vi "Command.vi"(8 "error in (no error)":errorcluster, 11 "Node Ptr":T1 format="%.0x") -> (0 "error out":errorcluster)   [LabVIEW 2018, in "Instrument Addon System Explorer.lvlib"]
uses:
  Instrument Addon System Explorer.lvlib
  <vilib>/NI Veristand/Custom Device API/Custom Device Item Ref.ctl
  APIs/Scripting API/TypeDefs/Command Settings.ctl
  APIs/Scripting API/TypeDefs/Padding.ctl
  APIs/Scripting API/TypeDefs/Linked Channel.ctl
  Addon Shared/Types/Linked Channel Cluster.ctl
  Addon Shared/SubVIs/Constants.vi
  <vilib>/Utility/file.llb/Write Delimited Spreadsheet (string).vi
  <vilib>/NI VeriStand/Custom Device API/Custom Device API.lvlib
  Addon Shared/Instrument Addon Shared.lvlib
  APIs/Scripting API/Instrument Addon Scripting API.lvlib
panel:
  in  "Pad Value":u8=32 format="%.0x"
  in  "Length":u32=25 caption="Length (Bytes)"
  in  "Pad":bool caption="Pad?"
  in  "Linkages":i32(listbox)
  in  "MetaData":string(combo) caption="Available MetaData Channels"
  in  "Command":string caption="Command ( Use [] to define a variable )"
  in  "Header 2":cluster{"Section Name":string}={"Section Name"="Command Message Settings"}
  in  "SHDocVw.IWebBrowser":refnum<k7>(container)
  in  "Header":cluster{"Section Name":string}={"Section Name"="Command Settings"}
  in  "Description":string
  out "Name":string
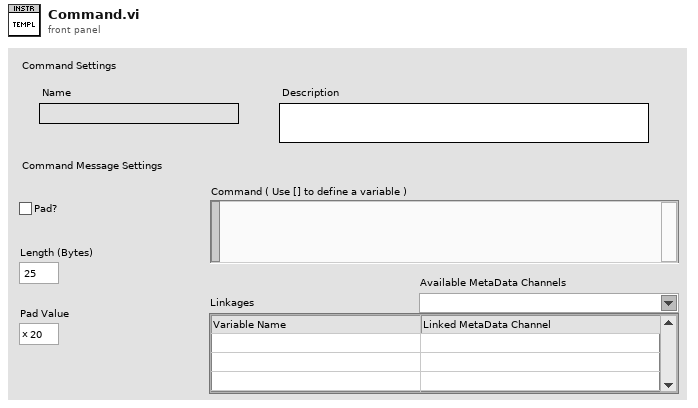
[diagram p1: front panel]
types:
  T1 = typedef "Custom Device API.lvlib/Custom Device Item Ref.ctl" = u64
  T2 = typedef "Instrument Addon Scripting API.lvlib/Command Settings.ctl" = cluster{"Command Format":string, "Use Padding?":bool, "Padding":T3, "Linkages":T4}
  T3 = typedef "Instrument Addon Scripting API.lvlib/Padding.ctl" = cluster{"Length":u32, "Pad Value":u8}
  T4 = typedef "Instrument Addon Scripting API.lvlib/Linked Channel.ctl" = cluster{"Channel Ref":T1, "Variable Name":string}[]
  T5 = typedef "Instrument Addon Shared.lvlib/Linked Channel Cluster.ctl" = cluster{"Variable Name":string, "GUID":string}
  T6 = cluster{"Channel Ref":T1, "Variable Name":string}
  T7 = typedef "Custom Device API.lvlib/Custom Device Item Info.ctl" = cluster{"Name":string, "Is Channel":bool, "GUID":string, "Is Waveform":bool}
  T8 = typedef "Custom Device API.lvlib/Custom Device Commands.ctl" = enum16{"Default", "Item renamed", "Shutdown", "Dynamic button pressed"}
  T9 = typedef "LVComboBoxStrsAndValuesArrayTypeDef.ctl" = cluster{"String":string, "Value":string}[]
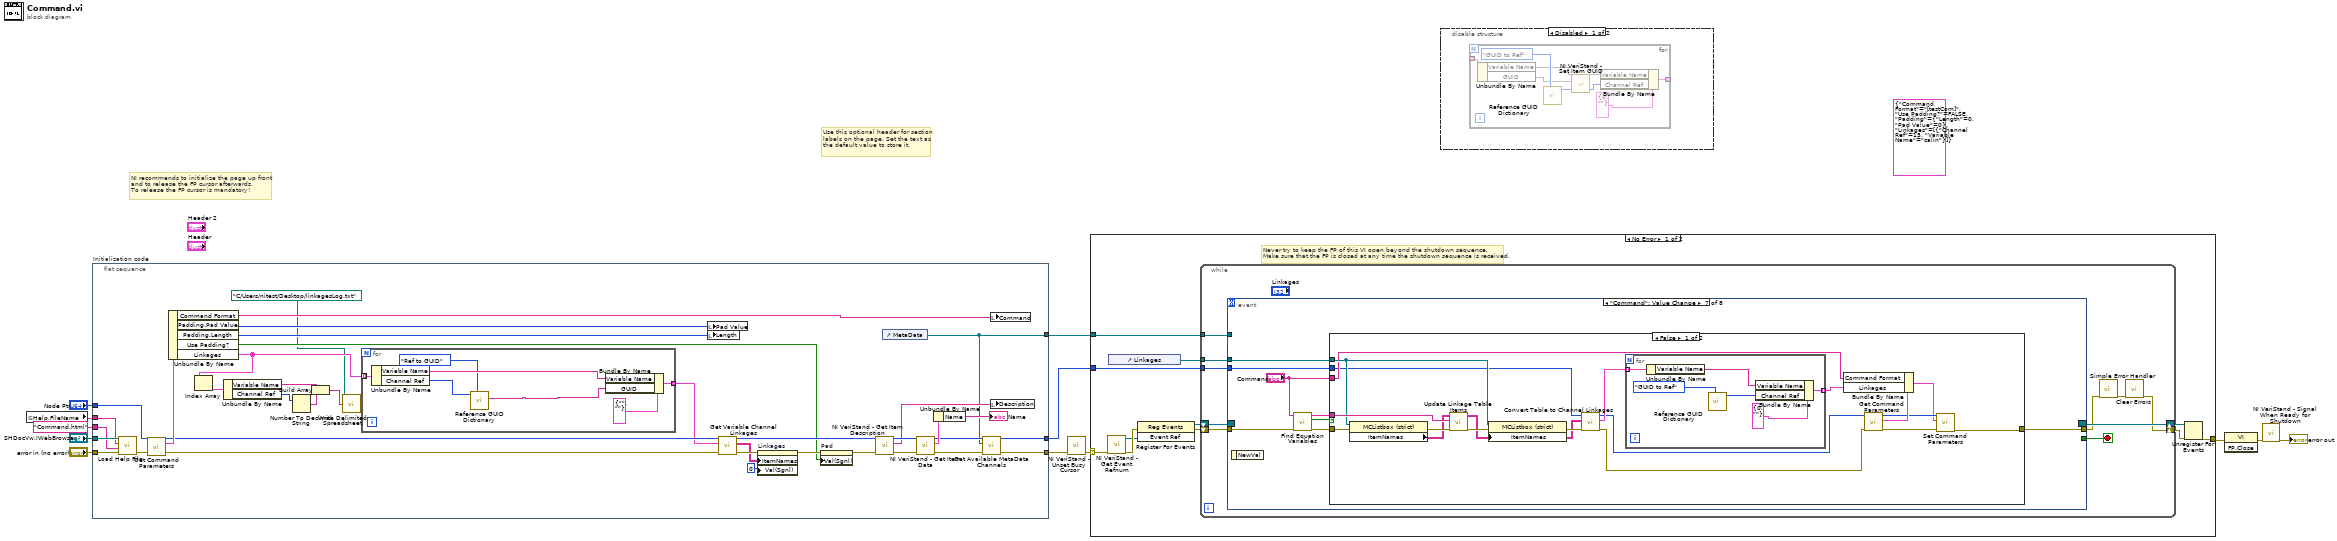
[diagram p0: block diagram]
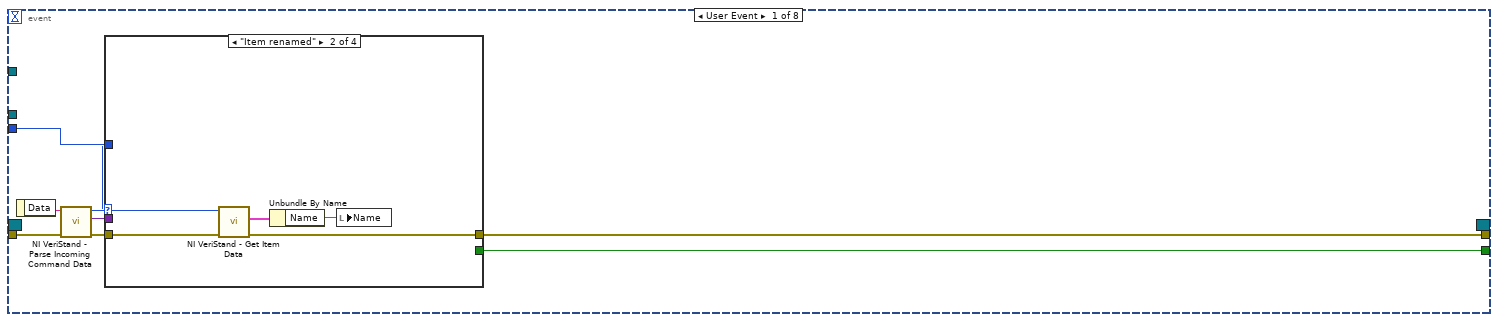
[diagram p3: hidden frame]
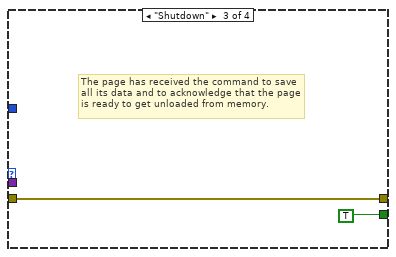
[diagram p5: hidden frame]
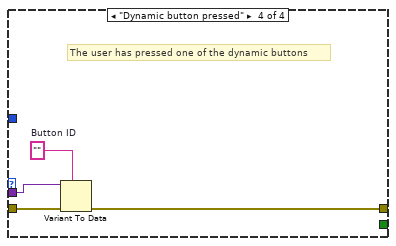
[diagram p6: hidden frame]
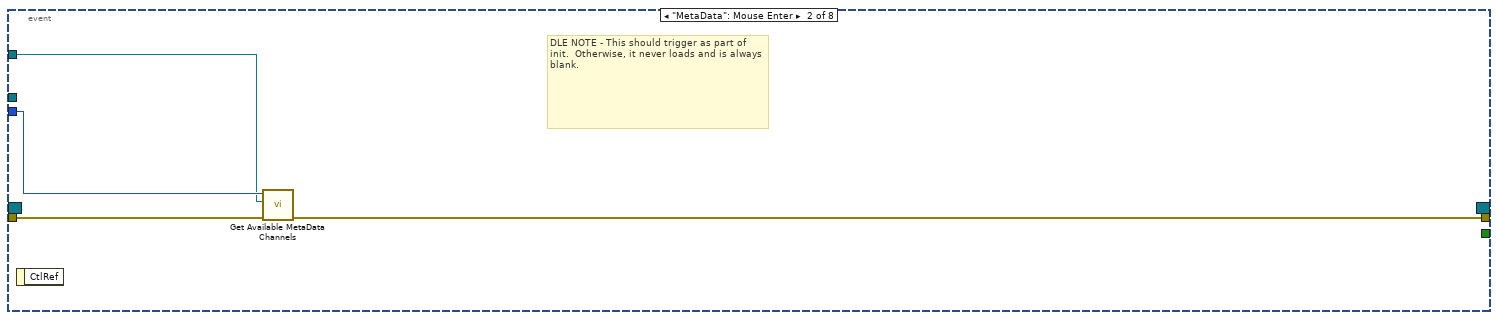
[diagram p7: hidden frame]
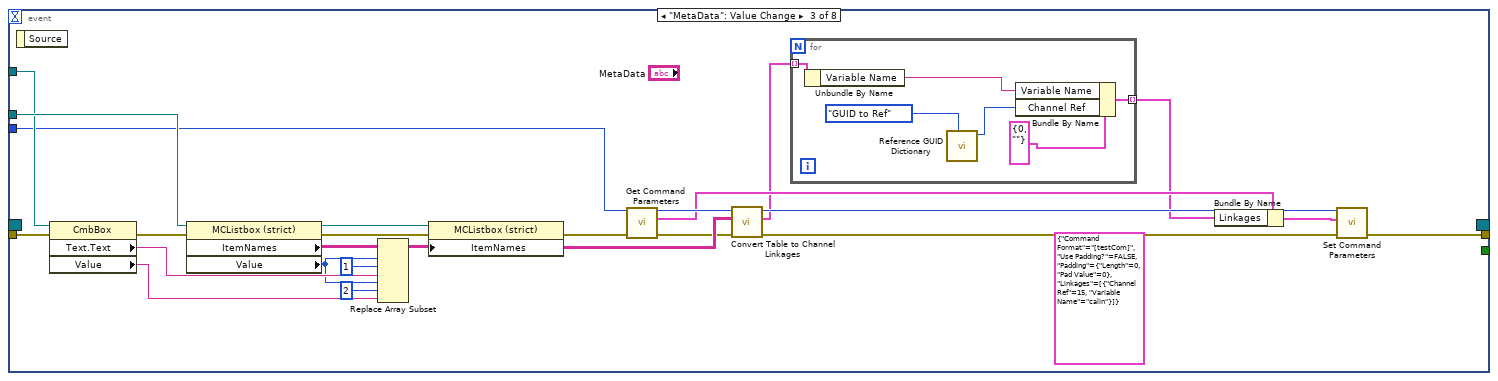
[diagram p8: hidden frame]
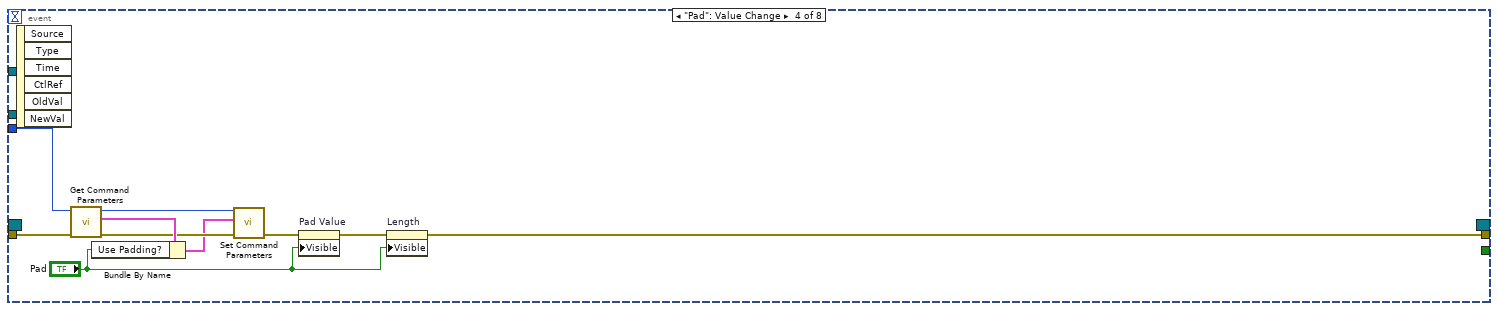
[diagram p9: hidden frame]
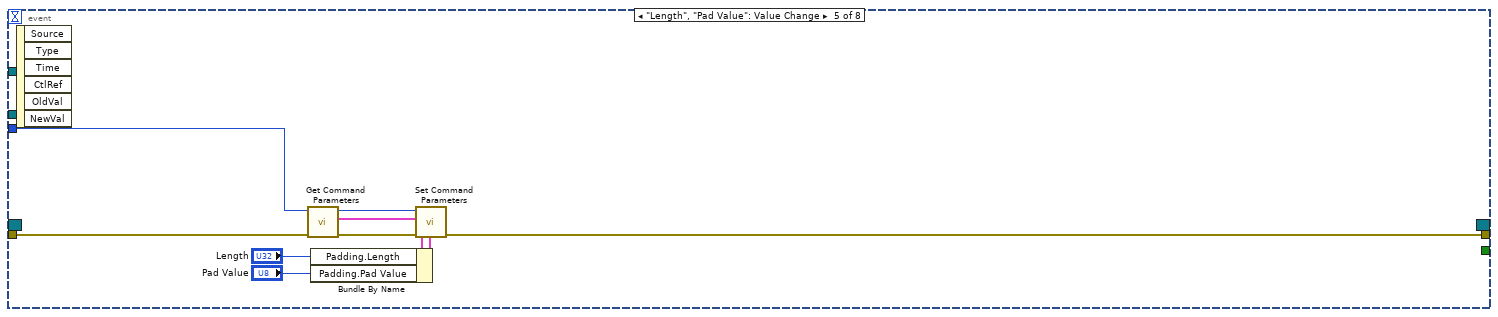
[diagram p10: hidden frame]
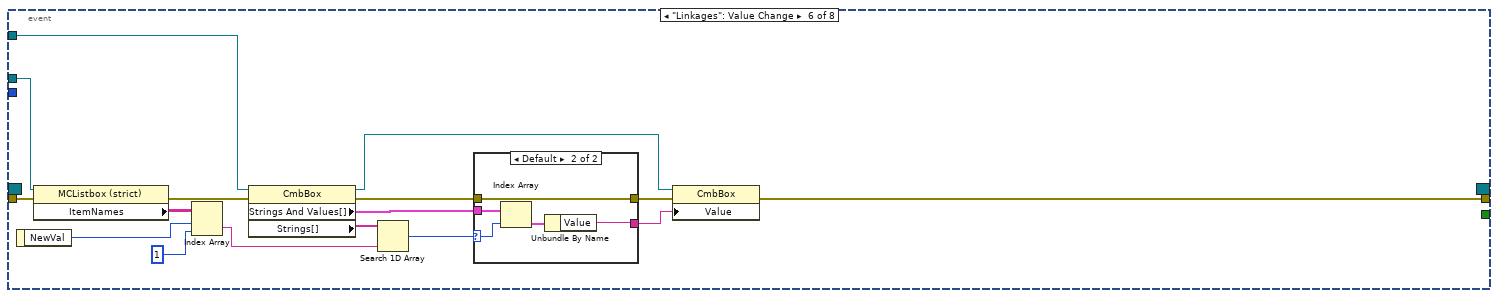
[diagram p11: hidden frame]
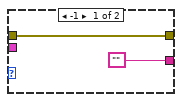
[diagram p12: hidden frame]
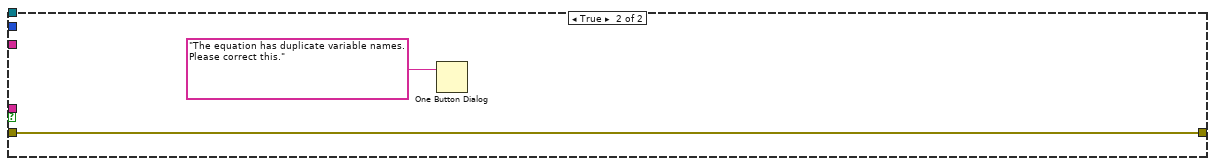
[diagram p13: hidden frame]
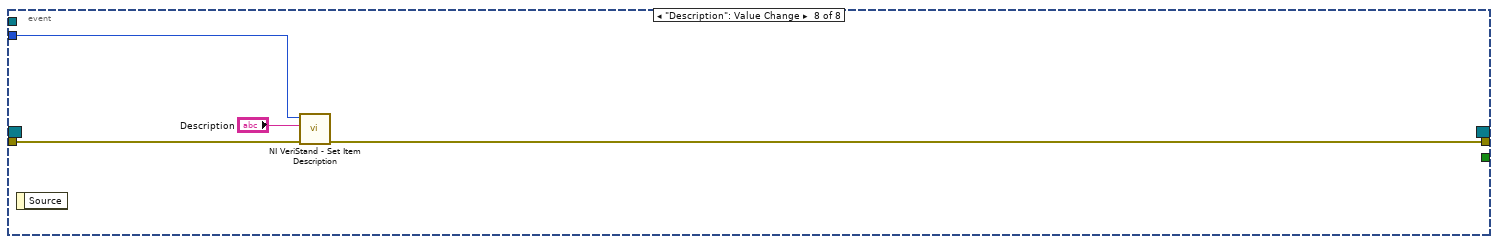
[diagram p14: hidden frame]
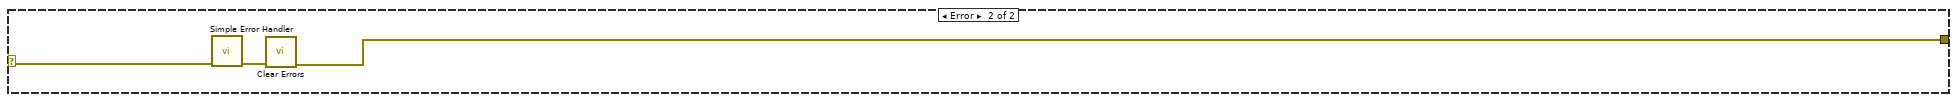
[diagram p15: hidden frame]
diagram:
  (unwired) T2 {"Command Format"="[testCom]", "Use Padding?"=FALSE, "Padding"={"Length"=0, "Pad Value"=0}, "Linkages"=[{"Channel Ref"=15, "Variable Name"="calin"}]} ("output cluster")
  # "Use this optional header for section labels on the page. Set the text as the default value to store it."
  # "NI recommends to initialize the page up front\nand to release the FP cursor afterwards.\nTo release the FP cursor is mandatory!"
  n1 = global read "Constants.vi" "Help.FileName"() -> (w1:string)
  n2 = flat-sequence "Initialization code" {
    tunnel: "error in (no error)" -> [w45]
    tunnel: "Node Ptr" -> [w26]
    tunnel: [w38] -> w8
    tunnel: [w36] -> w5
    tunnel: "SHDocVw.IWebBrowser" -> [w44]
    tunnel: "Command.html" ("HTML File") -> [w43]
    tunnel: w1 -> [w42]
    tunnel: [w20] -> w2
    frame #0 {
      n3 = call "Load Help File.vi"("error in (no error)"=w45, "HTML File"=w43, "Main CHM File"=w42, "SHDocVw.IWebBrowser2"=w44) -> ("error out"=w25:errorcluster)  [unwired: 7 in]
      n4 = call "Get Command Parameters.vi"("error in (no error)"=w25, "Item Ref in"=w26) -> ("error out"=w22:errorcluster, "Command Parameters Out"=w24:T2, "Item Ref out"=w23:T1)  [unwired: 7 in]
      n5 = Unbundle By Name(w24) -> ("Command Format"=w41:string, "Padding.Pad Value"=w28:u8, "Padding.Length"=w27:u32, "Use Padding?"=w29:bool, "Linkages"=w19:T4)
      n6 = Index Array(array=w19) -> (element=w18:T6)  [unwired: 1 in]
      n7 = Unbundle By Name(w18) -> ("Variable Name"=w15:string, "Channel Ref"=w17:T1)
      n8 = Number To Decimal String(number=w17) -> (decimal integer string=w16:string)  [unwired: 1 in]
      n9 = Build Array(w15, w16) -> (w14:string[])
      n10 = call-poly <vilib>:"Write Delimited Spreadsheet.vi"("file path (dialog if empty)"=path "C:/Users/nitest/Desktop/linkagesLog.txt", "1D data"=w14) -> ()  [unwired: 12 in, 2 out]
      n11 = for {
        tunnel: w19 -> [w56] mode=indexing
        tunnel: [w54] -> w21 mode=indexing
        n12 = Unbundle By Name(w56) -> ("Variable Name"=w53:string, "Channel Ref"=w52:T1)
        n13 = call "Reference GUID Dictionary.vi"("Enum"=enum16{"Ref to GUID", "GUID to Ref"}."Ref to GUID", "Channel Ref"=w52) -> ("GUID"=w50:string)  [unwired: 7 in, 2 out]
        n14 = Bundle By Name(cluster=T5 {"Variable Name"="", "GUID"=""} ("Linked Channel"), "Variable Name"=w53, "GUID"=w50) -> (w54:T5)
      }
      n15 = local write "Pad Value"(w28) -> ()
      n16 = local write "Length"(w27) -> ()
      n17 = call "Get Variable Channel Linkages.vi"("error in (no error)"=w22, "Linked Channels"=w21, "Item Ref in"=w23) -> ("error out"=w34:errorcluster, "Array"=w33:string[][], "Item Ref out"=w32:T1)  [unwired: 6 in]
      n18 = property on="Linkages" class="MCListbox (strict)"(error in=w34, "ItemNames"=w33, "Val(Sgnl)"=0 ("Value (Signaling)")) -> (error out=w31:errorcluster)  [unwired: 1 in, 1 out]
      n19 = property on="Pad" class="Bool (strict)"(error in=w31, "Val(Sgnl)"=w29) -> (error out=w30:errorcluster)  [unwired: 1 in, 1 out]
      n20 = call <vilib>:"NI VeriStand - Get Item Description.vi"("error in (no error)"=w30, "Item Ref in"=w32) -> ("error out"=w47:errorcluster, "Description"=w48:string, "Item Ref out"=w49:T1)  [unwired: 7 out]
      n21 = control-ref of="MetaData"() -> (w20:refnum<vi>)
      n22 = call <vilib>:"NI VeriStand - Get Item Data.vi"("error in (no error)"=w47, "Item Ref in"=w49) -> ("error out"=w39:errorcluster, "Item Info"=w46:T7, "Item Ref out"=w37:T1)  [unwired: 7 out]
      n23 = Unbundle By Name(w46) -> ("Name"=→"Name":string)
      n24 = call "Get Available MetaData Channels.vi"("error in (no error)"=w39, "Command"=w20, "Item Ref in"=w37) -> ("error out"=w38:errorcluster, "Item Ref out"=w36:T1)  [unwired: 7 in]
      n25 = local write "Command"(w41) -> ()
      n26 = local write "Description"(w48) -> ()
    }
  }
  n27 = call <vilib>:"NI VeriStand - Unset Busy Cursor.vi"("error in (no error)"=w8) -> ("error out"=w7:errorcluster)  [unwired: 10 out]
  n28 = case shown="No Error" w7 {
    selector: w7 -> [w59 w215]
    tunnel: [w64 w213] -> w12
    tunnel: w5 -> [w60 _]
    tunnel: w2 -> [w57 _]
    frame No Error {
      # "Never try to keep the FP of this VI open beyond the shutdown sequence.\nMake sure that the FP is closed at any time the shutdown sequence is received."
      n29 = call <vilib>:"NI VeriStand - Get Event Refnum.vi"("error in (no error)"=w59) -> ("error out"=w67:errorcluster, "Event Ref"=w63:refnum<user-event>)  [unwired: 9 out]
      n30 = control-ref of="Linkages"() -> (w58:refnum<vi>)
      n31 = register-events(error in=w67, w63) -> (reference out=w61:refnum<event-registration>, error out=w62:errorcluster)  [unwired: 1 in]
      n32 = while {
        tunnel: w60 -> [w69]
        shift-right: [w72] -> w65
        shift-left: w62 -> [w76]
        shift-right: [w77] -> w66
        shift-left: w61 -> [w75]
        tunnel: w58 -> [w71]
        tunnel: w57 -> [w70]
        stop <- w74 stop-if-true
        n33 = event shown="[6] \"Command\": Value Change" {
          selector: w75 -> [_ _ _ _ _ _ _ _]
          dyn-events: [_ _ _ _ _ _ _ _] -> w77
          timeout: _ -> [_ _ _ _ _ _ _ _]
          tunnel: w76 -> [w85 w101 w118 w139 w147 w166 w180 w211]
          tunnel: [w81 _ _ _ _ _ _ _] -> w74
          tunnel: [w80 w100 w106 w140 w142 w156 w177 w210] -> w68
          tunnel: w71 -> [_ _ w125 _ _ w165 w178 _]
          tunnel: w70 -> [_ w98 w119 _ _ w161 _ _]
          tunnel: w69 -> [w79 w99 w103 w138 w148 _ w175 w212]
          event User Event {
            n34 = event-data() -> ("Data"=w84:string)  [unwired: 1 out]
            n35 = call <vilib>:"NI VeriStand - Parse Incoming Command Data.vi"("error in (no error)"=w85, "Incoming data"=w84) -> ("error out"=w83:errorcluster, "Outgoing data"=w78:variant, "Action"=w82:T8)  [unwired: 7 out]
            n36 = case shown="\"Item renamed\"" w82 {
              tunnel: w83 -> [w86 w91 w92 w97]
              tunnel: [_ _ TRUE _] -> w81
              tunnel: [w86 w88 w92 w94] -> w80
              tunnel: w79 -> [_ w90 _ _]
              tunnel: w78 -> [_ _ _ w96]
              frame "Default", Default {
              }
              frame "Item renamed" {
                n37 = call <vilib>:"NI VeriStand - Get Item Data.vi"("error in (no error)"=w91, "Item Ref in"=w90) -> ("error out"=w88:errorcluster, "Item Info"=w89:T7)  [unwired: 8 out]
                n38 = Unbundle By Name(w89) -> ("Name"=w87:string)
                n39 = local write "Name"(w87) -> ()
              }
              frame "Shutdown" {
                # "The page has received the command to save all its data and to acknowledge that the page is ready to get unloaded from memory."
              }
              frame "Dynamic button pressed" {
                w95 = ""  # Button ID
                # "The user has pressed one of the dynamic buttons"
                n40 = Variant To Data(error in=w97, type=w95, Variant=w96) -> (error out=w94:errorcluster)  [unwired: 1 out]
              }
            }
          }
          event "MetaData": Mouse Enter {
            # "DLE NOTE - This should trigger as part of init.  Otherwise, it never loads and is always blank."
            n41 = event-data() -> ()  [unwired: 2 out]
            n42 = call "Get Available MetaData Channels.vi"("error in (no error)"=w101, "Command"=w98, "Item Ref in"=w99) -> ("error out"=w100:errorcluster)  [unwired: 7 in, 1 out]
          }
          event "MetaData": Value Change {
            (unwired) T2 {"Command Format"="[testCom]", "Use Padding?"=FALSE, "Padding"={"Length"=0, "Pad Value"=0}, "Linkages"=[{"Channel Ref"=15, "Variable Name"="calin"}]} ("output cluster")
            n43 = event-data() -> ()  [unwired: 2 out]
            n44 = property class="CmbBox"(reference=w119, error in=w118) -> (error out=w117:errorcluster, "Text.Text"=w116:string, "Value"=w114:string)  [unwired: 1 out]
            n45 = property class="MCListbox (strict)"(reference=w125, error in=w117) -> (reference out=w122:refnum<vi>, error out=w121:errorcluster, "ItemNames"=w124:string[][], "Value"=w115:i32)
            n46 = Replace Array Subset(array=w124, new element #1=w116, index (row) #1=w115, index (col) #1=1 ("disabled index (col)"), new element #2=w114, index (row) #2=w115, index (col) #2=2 ("disabled index (col)")) -> (w113:string[][])
            n47 = property class="MCListbox (strict)"(reference=w122, error in=w121, "ItemNames"=w113) -> (error out=w112:errorcluster)  [unwired: 1 out]
            n48 = call "Get Command Parameters.vi"("error in (no error)"=w112, "Item Ref in"=w103) -> ("error out"=w110:errorcluster, "Command Parameters Out"=w109:T2, "Item Ref out"=w111:T1)  [unwired: 7 in]
            n49 = call "Convert Table to Channel Linkages.vi"("error in (no error)"=w110, "Item Names"=w113, "Item Ref in"=w111) -> ("error out"=w108:errorcluster, "Linkages"=w105:T5[], "Item Ref out"=w107:T1)  [unwired: 6 in]
            n50 = for {
              tunnel: w105 -> [w131] mode=indexing
              tunnel: [w129] -> w104 mode=indexing
              n51 = Unbundle By Name(w131) -> ("Variable Name"=w130:string)
              n52 = call "Reference GUID Dictionary.vi"("Enum"=enum16{"Ref to GUID", "GUID to Ref"}."GUID to Ref") -> ("Channel Ref Out"=w126:T1)  [unwired: 8 in, 2 out]
              n53 = Bundle By Name(cluster=T6 {"Channel Ref"=0, "Variable Name"=""} ("element"), "Variable Name"=w130, "Channel Ref"=w126) -> (w129:T6)
            }
            n54 = Bundle By Name(cluster=w109, "Linkages"=w104) -> (w102:T2)
            n55 = call "Set Command Parameters.vi"("error in (no error)"=w108, "Command Parameters In"=w102, "Item Ref in"=w107) -> ("error out"=w106:errorcluster)  [unwired: 6 in, 2 out]
          }
          event "Pad": Value Change {
            n56 = event-data() -> ()  [unwired: 7 out]
            n57 = call "Get Command Parameters.vi"("error in (no error)"=w139, "Item Ref in"=w138) -> ("error out"=w135:errorcluster, "Command Parameters Out"=w137:T2, "Item Ref out"=w136:T1)  [unwired: 7 in]
            n58 = Bundle By Name(cluster=w137, "Use Padding?"="Pad") -> (w133:T2)
            n59 = call "Set Command Parameters.vi"("error in (no error)"=w135, "Command Parameters In"=w133, "Item Ref in"=w136) -> ("error out"=w134:errorcluster)  [unwired: 6 in, 2 out]
            n60 = property on="Pad Value" class="DigNum (strict)"(error in=w134, "Visible"="Pad") -> (error out=w141:errorcluster)  [unwired: 1 in, 1 out]
            n61 = property on="Length" class="DigNum (strict)"(error in=w141, "Visible"="Pad") -> (error out=w140:errorcluster)  [unwired: 1 in, 1 out]
          }
          event "Length", "Pad Value": Value Change {
            n62 = event-data() -> ()  [unwired: 7 out]
            n63 = call "Get Command Parameters.vi"("error in (no error)"=w147, "Item Ref in"=w148) -> ("error out"=w143:errorcluster, "Command Parameters Out"=w146:T2, "Item Ref out"=w144:T1)  [unwired: 7 in]
            n64 = Bundle By Name(cluster=w146, "Padding.Length"="Length", "Padding.Pad Value"="Pad Value") -> (w145:T2)
            n65 = call "Set Command Parameters.vi"("error in (no error)"=w143, "Command Parameters In"=w145, "Item Ref in"=w144) -> ("error out"=w142:errorcluster)  [unwired: 6 in, 2 out]
          }
          event "Linkages": Value Change {
            n66 = event-data() -> ("NewVal"=w163:i32)  [unwired: 1 out]
            n67 = property class="MCListbox (strict)"(reference=w165, error in=w166) -> (error out=w160:errorcluster, "ItemNames"=w164:string[][])  [unwired: 1 out]
            n68 = Index Array(array=w164, index (row)=w163, index (col)=1 ("disabled index (col)")) -> (element=w159:string)
            n69 = property class="CmbBox"(reference=w161, error in=w160) -> (reference out=w154:refnum<vi>, error out=w152:errorcluster, "Strings And Values[]"=w158:T9, "Strings[]"=w151:string[])
            n70 = Search 1D Array(1D array=w151, element=w159) -> (index of element=w155:i32)  [unwired: 1 in]
            n71 = case shown="Default" w155 {
              selector: w155 -> [_ w171]
              tunnel: w158 -> [_ w173]
              tunnel: ["" w169] -> w157
              tunnel: [w168 w170] -> w153
              tunnel: w152 -> [w168 w170]
              frame -1 {
              }
              frame Default {
                n72 = Index Array(array=w173, index=w171) -> (element=w172:cluster{"String":string, "Value":string})
                n73 = Unbundle By Name(w172) -> ("Value"=w169:string)
              }
            }
            n74 = property class="CmbBox"(reference=w154, error in=w153, "Value"=w157) -> (error out=w156:errorcluster)  [unwired: 1 out]
          }
          event "Command": Value Change {
            n75 = event-data() -> ()  [unwired: 2 out]
            n76 = call "Find Equation Variables.vi"("error in (no error)"=w180, "Command"="Command") -> ("error out"=w179:errorcluster, "Duplicate?"=w174:bool, "Variables"=w181:string[])  [unwired: 7 in]
            n77 = case shown="False" w174 {
              tunnel: w181 -> [w200 _]
              tunnel: w179 -> [w199 w208]
              tunnel: w178 -> [w195 _]
              tunnel: [w187 w208] -> w177
              tunnel: "Command" -> [w194 _]
              tunnel: w175 -> [w183 _]
              frame False {
                n78 = property class="MCListbox (strict)"(reference=w195, error in=w199) -> (error out=w198:errorcluster, "ItemNames"=w197:string[][])  [unwired: 1 out]
                n79 = call "Update Linkage Table Items.vi"("error in (no error)"=w198, "Variables"=w200, "Item Names"=w197) -> ("error out"=w196:errorcluster, "Item Names"=w192:string[][])  [unwired: 7 in]
                n80 = property class="MCListbox (strict)"(reference=w195, error in=w196, "ItemNames"=w192) -> (error out=w193:errorcluster)  [unwired: 1 out]
                n81 = call "Convert Table to Channel Linkages.vi"("error in (no error)"=w193, "Item Names"=w192, "Item Ref in"=w183) -> ("error out"=w191:errorcluster, "Linkages"=w186:T5[], "Item Ref out"=w182:T1)  [unwired: 6 in]
                n82 = for {
                  tunnel: w186 -> [w206] mode=indexing
                  tunnel: [w204] -> w185 mode=indexing
                  n83 = Unbundle By Name(w206) -> ("Variable Name"=w205:string)
                  n84 = call "Reference GUID Dictionary.vi"("Enum"=enum16{"Ref to GUID", "GUID to Ref"}."GUID to Ref") -> ("Channel Ref Out"=w202:T1)  [unwired: 8 in, 2 out]
                  n85 = Bundle By Name(cluster=T6 {"Channel Ref"=0, "Variable Name"=""} ("Linkages"), "Variable Name"=w205, "Channel Ref"=w202) -> (w204:T6)
                }
                n86 = call "Get Command Parameters.vi"("error in (no error)"=w191, "Item Ref in"=w182) -> ("error out"=w189:errorcluster, "Command Parameters Out"=w190:T2, "Item Ref out"=w188:T1)  [unwired: 7 in]
                n87 = Bundle By Name(cluster=w190, "Command Format"=w194, "Linkages"=w185) -> (w184:T2)
                n88 = call "Set Command Parameters.vi"("error in (no error)"=w189, "Command Parameters In"=w184, "Item Ref in"=w188) -> ("error out"=w187:errorcluster)  [unwired: 6 in, 2 out]
              }
              frame True {
                n89 = One Button Dialog(message="The equation has duplicate variable names.  Please correct this.") -> ()  [unwired: 1 in, 1 out]
              }
            }
          }
          event "Description": Value Change {
            n90 = event-data() -> ()  [unwired: 2 out]
            n91 = call <vilib>:"NI VeriStand - Set Item Description.vi"("error in (no error)"=w211, "Description"="Description", "Item Ref in"=w212) -> ("error out"=w210:errorcluster)  [unwired: 8 out]
          }
        }
        n92 = call <vilib>:"Simple Error Handler.vi"("error in (no error)"=w68) -> ("error out"=w73:errorcluster)  [unwired: 1 in, 7 out]
        n93 = call <vilib>:"Clear Errors.vi"("error in (no error)"=w73) -> ("error out"=w72:errorcluster)  [unwired: 1 in, 5 out]
      }
      n94 = Unregister For Events(event registration refnum=w66, error in=w65) -> (error out=w64:errorcluster)
    }
    frame Error {
      n95 = call <vilib>:"Simple Error Handler.vi"("error in (no error)"=w215) -> ("error out"=w214:errorcluster)  [unwired: 1 in, 7 out]
      n96 = call <vilib>:"Clear Errors.vi"("error in (no error)"=w214) -> ("error out"=w213:errorcluster)  [unwired: 1 in, 5 out]
    }
  }
  n97 = disable-structure shown="Disabled" {
    frame Disabled {
      n98 = for {
        tunnel: _ -> [w222] mode=indexing
        tunnel: [w219] -> _ mode=indexing
        n99 = Unbundle By Name(w222) -> ("Variable Name"=w220, "GUID"=w216)
        n100 = call "Reference GUID Dictionary.vi"("Enum"=enum16{"Ref to GUID", "GUID to Ref"}."GUID to Ref") -> ("Channel Ref Out"=w218:T1)  [unwired: 8 in, 2 out]
        n101 = call <vilib>:"NI VeriStand - Set Item GUID.vi"("GUID"=w216) -> ()  [unwired: 9 in, 2 out]
        n102 = Bundle By Name(cluster=T6 {"Channel Ref"=0, "Variable Name"=""} ("element"), "Variable Name"=w220, "Channel Ref"=w218) -> (w219:T6)
      }
    }
    frame Enabled {
    }
  }
  n103 = invoke class="VI" method="FP.Close"(error in=w12) -> (error out=w11:errorcluster)  [unwired: 2 in, 2 out]
  n104 = call <vilib>:"NI VeriStand - Signal When Ready for Shutdown.vi"("error in (no error)"=w11) -> ("error out"=→"error out":errorcluster)  [unwired: 10 out]
